vi "Default Settings.vi"(8 "error in (no error)":errorcluster, 11 "Crosshair Dispense in":refnum<class "Crosshair Dispense.lvclass">) -> (0 "error out":errorcluster, 3 "Crosshair Dispense out":refnum<class "Crosshair Dispense.lvclass">)   [LabVIEW 2019, in "Crosshair Dispense.lvclass"]
uses:
  Crosshair Dispense.lvclass
  C:/Users/HEP/Documents/Aerotech gantry/UCSB-Gantry-master-main/V5/Classes/Routine/Dispense/Dispense.lvclass
  Crosshair Dispense.lvclass/Crosshair Dispense.ctl
  Dispense.lvclass/Dispense.ctl
  Write Tip Height.vi
  Dispense.lvclass
panel:
  # "This Routine does not Accept Settings"
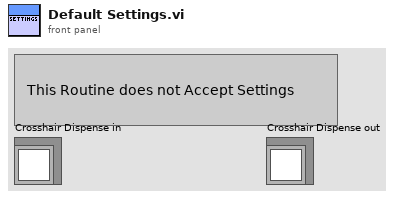
[diagram p1: front panel]
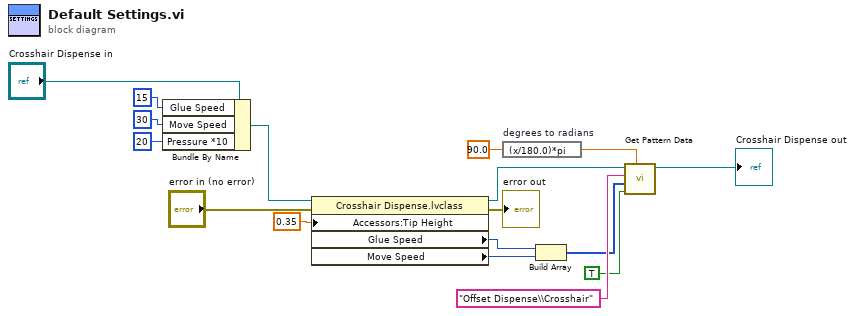
[diagram p0: block diagram]
diagram:
  n1 = Bundle By Name(cluster="Crosshair Dispense in", "Glue Speed"=15, "Move Speed"=30, "Pressure *10"=i64 20) -> (w17:refnum<class "Crosshair Dispense.lvclass">)
  n2 = property class="Crosshair Dispense.lvclass"(reference=w17, error in="error in (no error)", "Accessors:Tip Height"=0.35 ("Tip Height")) -> (reference out=w9:refnum<class "Crosshair Dispense.lvclass">, error out=→"error out":errorcluster, "Glue Speed"=w7:i32, "Move Speed"=w1:i32)
  n3 = expression code="(x/180.0)*pi" "degrees to radians"(90.0 ("theta")) -> (w4:dbl)
  n4 = Build Array(w7, w1) -> (w6:i32[])
  n5 = call "Get Pattern Data.vi"("theta"=w4, "Iterative?"=TRUE, "File Name"=w6, "Folder Name"="Offset Dispense\\Crosshair", "Dispense.lvclass"=w9) -> ("Dispense Out"=→"Crosshair Dispense out":refnum<class "Crosshair Dispense.lvclass">)  [unwired: 6 in]
